vi "Init.vi"(8 "error in":errorcluster) -> (0 "error out":errorcluster, 3 "Visa Array out":refnum<visa-resource-name>[](array[refnum]))   [LabVIEW 2010, in "SignalWriterMH110203USBStepperMotor.lvclass"]
uses:
  SignalWriterMH110203USBStepperMotor.lvclass
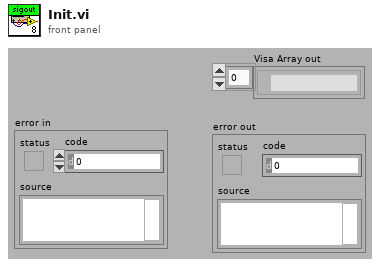
[diagram p1: front panel]
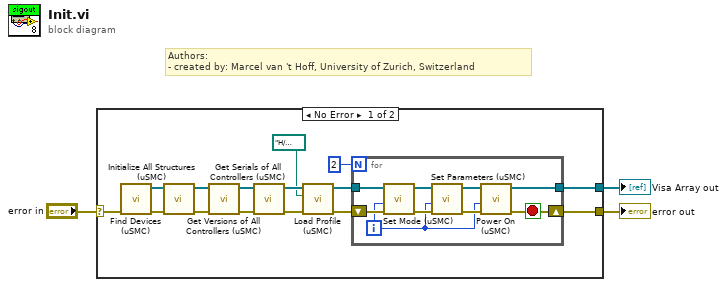
[diagram p0: block diagram]
diagram:
  # "Authors: \n- created by: Marcel van 't Hoff, University of Zurich, Switzerland"
  n1 = case shown="No Error" "error in" {
    selector: "error in" -> [w17 w28]
    tunnel: [w5 _] -> w1
    tunnel: [w4 w28] -> w3
    frame No Error {
      n2 = call "Find Devices (uSMC).vi"("error in (no error)"=w17) -> ("error out"=w11:errorcluster, "Visa array out"=w12:refnum<visa-resource-name>[])  [unwired: 8 in, 1 out]
      n3 = call "Initialize All Structures (uSMC).vi"("error in"=w11, "Visa array in"=w12) -> ("error out"=w15:errorcluster, "Visa array out"=w13:refnum<visa-resource-name>[])  [unwired: 8 in]
      n4 = call "Get Versions of All Controllers (uSMC).vi"("error in"=w15, "Visa array in"=w13) -> ("error out"=w16:errorcluster, "Visa array out"=w14:refnum<visa-resource-name>[])  [unwired: 7 in, 1 out]
      n5 = call "Get Serials of All Controllers (uSMC).vi"("error in (no error)"=w16, "Visa array in"=w14) -> ("error out"=w10:errorcluster, "Visa array out"=w8:refnum<visa-resource-name>[])  [unwired: 7 in, 1 out]
      n6 = call "Load Profile (uSMC).vi"("error in"=w10, "Path"=path "H:/Programming/+ Labview/10 uEye camera/100923/subVI/Standa/Standa_8MR151-1-670mA_D-Sub-15Pin.pre", "Visa array in"=w8) -> ("error out"=w9:errorcluster, "Visa array out"=w7:refnum<visa-resource-name>[])  [unwired: 6 in, 1 out]
      n7 = for {
        N: 2 -> [_]
        tunnel: [w20] -> w5
        tunnel: w7 -> [w23]
        shift-right: [w19] -> w4
        shift-left: w9 -> [w26]
        i -> [w21]
        stop <- w19 stop-if-true
        n8 = call "Set Mode (uSMC).vi"("error in (no error)"=w26, "Index"=w21, "Visa Array in"=w23) -> ("error out"=w27:errorcluster, "Visa Array out"=w24:refnum<visa-resource-name>[])  [unwired: 7 in]
        n9 = call "Set Parameters (uSMC).vi"("error in (no error)"=w27, "Index"=w21, "Visa array in"=w24) -> ("error out"=w25:errorcluster, "Visa Array out"=w22:refnum<visa-resource-name>[])  [unwired: 7 in]
        n10 = call "Power On (uSMC).vi"("error in (no error)"=w25, "Index"=w21, "Visa Array in"=w22) -> ("error out"=w19:errorcluster, "Visa Array out"=w20:refnum<visa-resource-name>[])  [unwired: 7 in]
      }
    }
    frame Error {
    }
  }
  "Visa Array out" <- w1
  "error out" <- w3
